vi "LV BootCamp - Broken VI - for Students.vi"() -> ()   [LabVIEW 2016]
panel:
  in  "Input Temperature (deg C)":dbl(slide) scale=0.0..100.0
  out "In Range?":dbl
  out "Current Temperature (deg F)":dbl
  out "Current Temperature (deg C)":dbl
  in  "Lower  Limit (deg C)":dbl
  in  "Upper Limit (deg C)":dbl
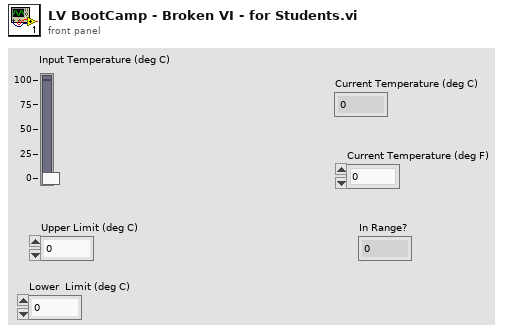
[diagram p1: front panel]
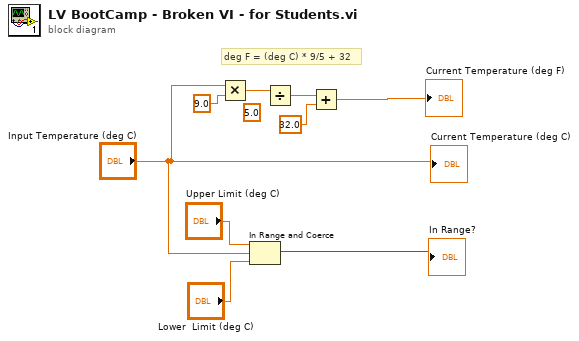
[diagram p0: block diagram]
diagram:
  (unwired) 5.0 ("y")
  # "deg F = (deg C) * 9/5 + 32"
  n1 = Multiply(x="Input Temperature (deg C)", y=9.0) -> (x*y=w9:dbl)
  n2 = In Range and Coerce(upper limit="Upper Limit (deg C)", x="Input Temperature (deg C)", lower limit="Lower  Limit (deg C)") -> (In Range?=→"In Range?":bool)  [unwired: 1 out]
  n3 = Divide(x=w9) -> (x/y=w8:dbl)  [unwired: 1 in]
  n4 = Add(x=w8, y=32.0) -> (x+y=→"Current Temperature (deg F)":dbl)
  "Current Temperature (deg C)" <- "Input Temperature (deg C)"
